vi "GEAHexToASCIIString.vi"(10 "GEA HEX":string="4E 52 54 52 4D 50 47 56 00 00 00 00 00 00 00 00 00 00 00 00 00 00 00 00 00 00 00 00 00 00 00 00") -> (2 "ASCII String":string)   [LabVIEW 2013]
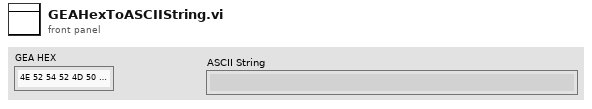
[diagram p1: front panel]
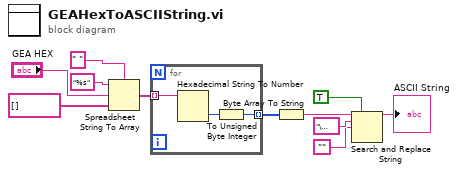
[diagram p0: block diagram]
diagram:
  n1 = Spreadsheet String To Array(delimiter (Tab)=" ", format string="%s", spreadsheet string="GEA HEX", array type (2D Dbl)=string[] []) -> (array=w7:string[])
  n2 = for {
    tunnel: w7 -> [w14] mode=indexing
    tunnel: [w12] -> w6 mode=indexing
    n3 = Hexadecimal String To Number(string=w14) -> (number=w13:u32)  [unwired: 2 in, 1 out]
    n4 = To Unsigned Byte Integer(number=w13) -> (unsigned 8bit integer=w12:u8)
  }
  n5 = Byte Array To String(unsigned byte array=w6) -> (string=w5:string)
  n6 = Search and Replace String(replace all?=TRUE ("replace all? (F)"), input string=w5, search string="\u0000", replace string="") -> (result string=→"ASCII String":string)  [unwired: 4 in, 3 out]
